vi "chaos crest reg time.vi"(11 "h":u32) -> (2 "function return":sgl, 3 "h out":u32)   [LabVIEW 2014, in "libcommon-crest.lvlib"]
doc: "float chaos_crest_reg_time(chaos_crest_handle_t h);"
uses:
  libcommon-crest.lvlib
  chaos-i686-dynamic-release/lib/libcommon-crest.so
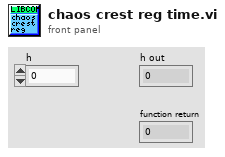
[diagram p1: front panel]
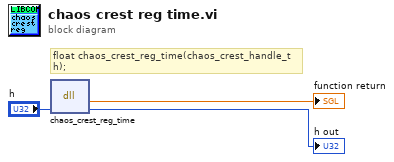
[diagram p0: block diagram]
diagram:
  # "float chaos_crest_reg_time(chaos_crest_handle_t h);"
  n1 = dll-call lib="home/chaos/chaos_bundle/chaos-i686-dynamic-release/lib/libcommon-crest.*" fn="chaos_crest_reg_time"("h"="h") -> (→"function return":sgl, "h"=→"h out":u32)  [unwired: 3 in, 2 out]
